vi "Change_Stack_New.vi"   [LabVIEW 2019]
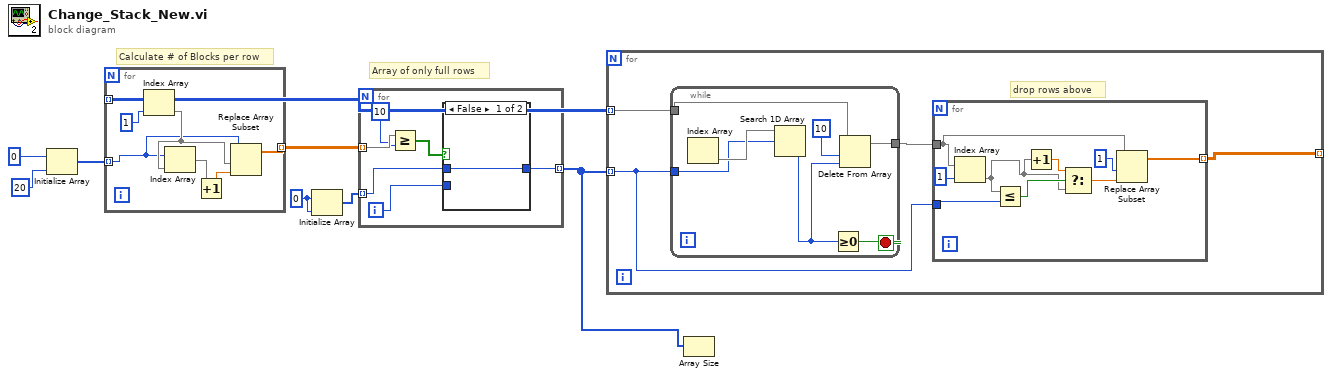
[diagram p0: block diagram]
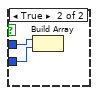
[diagram p2: hidden frame]
diagram:
  w6 = 0
  # "Array of only full rows"
  # "Calculate # of Blocks per row"
  n1 = Initialize Array(0, 20) -> (w7:i32[])
  n2 = for {
    tunnel: [w15] -> w2 mode=indexing
    tunnel: w7 -> [w10] mode=indexing
    tunnel: [w12] -> w5 mode=indexing
    n3 = Index Array(array=w15, index=1) -> (element=w11)
    n4 = Index Array(array=w10, index=w11) -> (element=w13)
    n5 = Increment(x=w13) -> (x+1=w14:dbl)
    n6 = Replace Array Subset(array=w10, new element=w14, index=w11) -> (w12:dbl[])
  }
  n7 = Initialize Array(w6, w6) -> (w4:i32[])
  n8 = for {
    tunnel: w5 -> [w22] mode=indexing
    tunnel: w4 -> [w20] mode=indexing
    tunnel: [w17] -> w3 mode=indexing
    i -> [w19]
    n9 = Greater Or Equal?(x=w22, y=10) -> (x >= y?=w18:bool[])
    n10 = case shown="False" w18 {
      tunnel: w20 -> [w23 w25]
      tunnel: w19 -> [_ w24]
      tunnel: [w23 _] -> w17
      frame False {
      }
      frame True {
        n11 = Build Array(w25, w24) -> ()  [unwired: 1 out]
      }
    }
  }
  n12 = for {
    tunnel: w3 -> [w28] mode=indexing
    tunnel: w2 -> [w29] mode=indexing
    tunnel: [w26] -> _ mode=indexing
    # "drop rows above"
    n13 = while {
      tunnel: w28 -> [w43]
      tunnel: w29 -> [w40]
      tunnel: [w39] -> w27
      stop <- w45 stop-if-true
      n14 = Index Array() -> (element=w44)  [unwired: 2 in]
      n15 = Search 1D Array(1D array=w44, element=w43) -> (index of element=w42:i32)  [unwired: 1 in]
      n16 = Greater Or Equal To 0?(x=w42) -> (x >= 0?=w45:bool)
      n17 = Delete From Array(array=w40, length=10, index=w42) -> (array with subset deleted=w39)  [unwired: 1 out]
    }
    n18 = for {
      tunnel: w28 -> [w37]
      tunnel: w27 -> [w30]
      tunnel: [w31] -> w26 mode=indexing
      n19 = Index Array(array=w30, index=1) -> (element=w34)
      n20 = Less Or Equal?(x=w34, y=w37) -> (x <= y?=w36:bool)
      n21 = Increment(x=w34) -> (x+1=w35:dbl)
      n22 = Select(t=w35, s=w36, f=w34) -> (s? t:f=w33:dbl)
      n23 = Replace Array Subset(array=w30, new element=w33, index=1) -> (w31:dbl[])
    }
  }
  n24 = Array Size(array=w3) -> (size(s)=w1:i32)
